vi "VisualizeWfrm.vi"() -> ()   [LabVIEW 2014, in "Visualization.lvlib" / "VisualizeWfrm.lvclass"]
uses:
  VisualizeWfrm.lvclass
  VisualizeBase/VisualizeBase_class/Requests/clUserEventType.ctl
  <vilib>/event_ctls.llb/usereventprio.ctl
  <vilib>/Utility/error.llb/Error Cluster From Error Code.vi
  <vilib>/ErrorRing/Error Ring.xnode
  VisualizeBase/VisualizeBase_class/VisualizeBase.lvclass
  <userlib>/NIST/NISTErrorLib/NISTErrorLib.lvlib
  WfrmGenerator/WfrmModule/WfrmModule.lvlib
panel:
  out "Currents":dbl[][](graph)
  out "Voltages":dbl[][](graph)
  in  "QueName":string="WfrmVisQue"
  out "ErrorArray":errorcluster[](array[cluster])
  in  "btnStop":bool
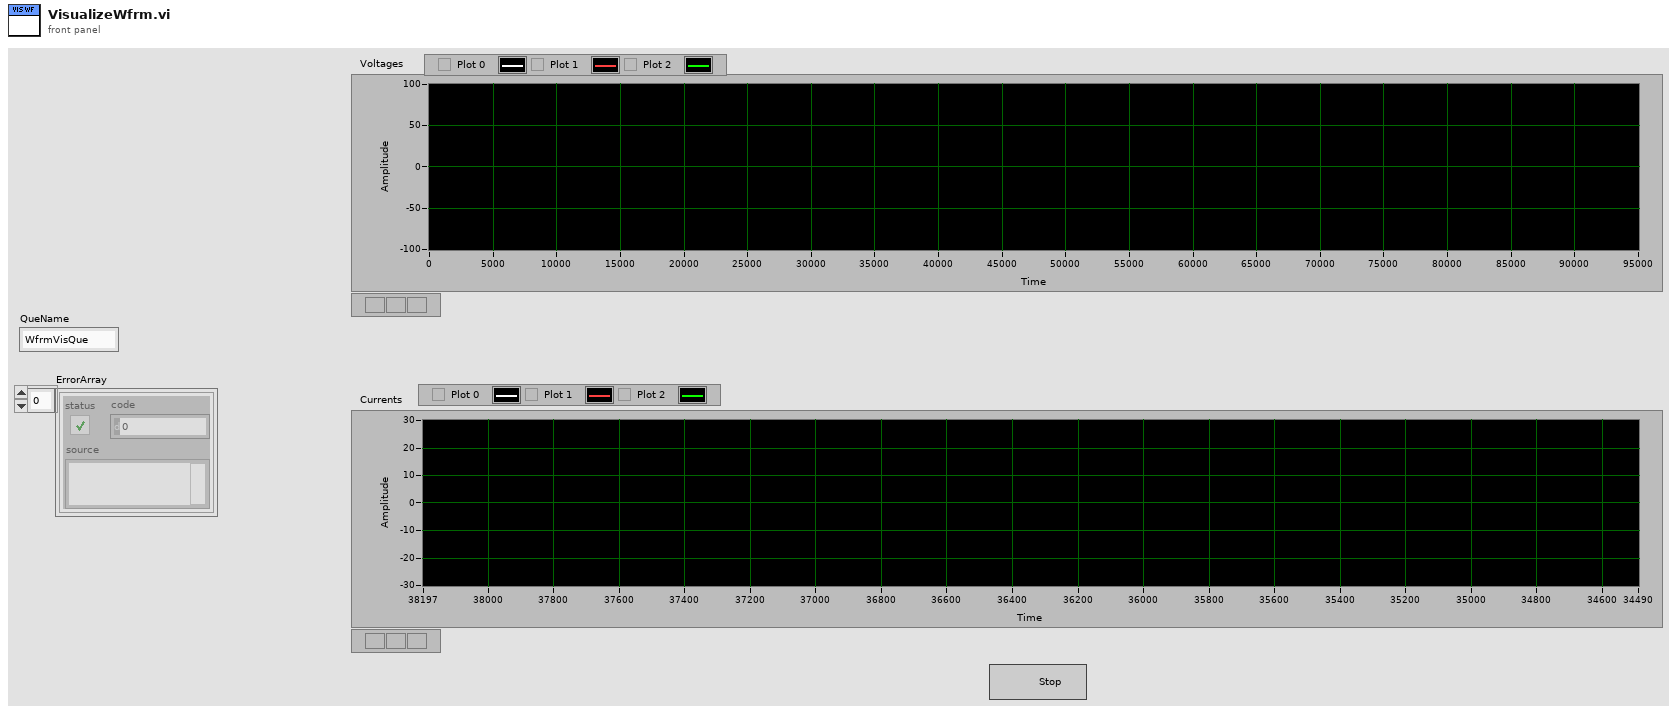
[diagram p1: front panel]
types:
  T1 = typedef "Visualization.lvlib/VisualizeBase.lvclass/clRequestEvents.ctl" = cluster{"StopRequest":refnum<user-event>}
  T2 = typedef "WfrmModule.lvlib/clBroadcastEvents.ctl" = cluster{"DidInit":refnum<user-event>, "StatusUpdate":refnum<user-event>, "ErrorReport":refnum<user-event>, "DidStop":refnum<user-event>, "ReadEvtConfig":refnum<user-event>, "ReadTimeArray":refnum<user-event>, "ReadEvtParams":refnum<user-event>, "GetEvtReportArray":refnum<user-event>, "ReadPathToPlugin":refnum<user-event>, "GetEvtSignal":refnum<user-event>, "SendArbWfrm":refnum<user-event>, "WfrmParams":refnum<user-event>}
  T3 = typedef "Visualization.lvlib/VisualizeBase.lvclass/clUserEventType.ctl" = cluster{"BusIndex":i8, "Data":variant}
  T4 = typedef "usereventprio.ctl" = enum32{"high priority", "normal priority"}
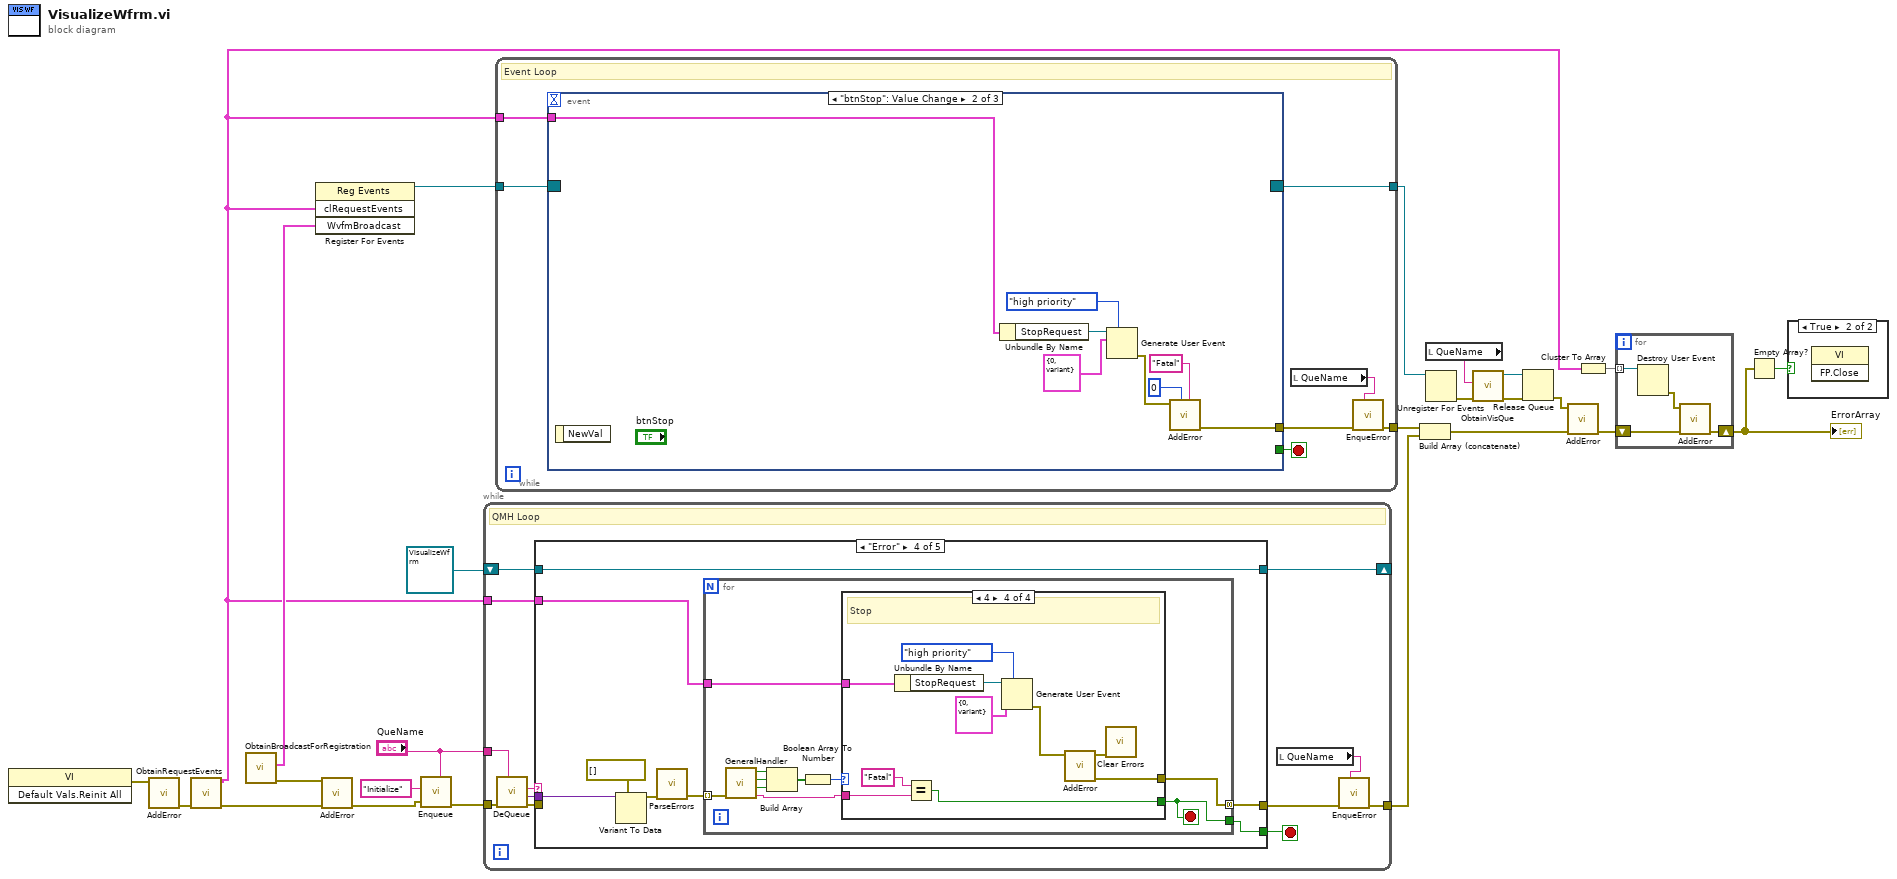
[diagram p0: block diagram]
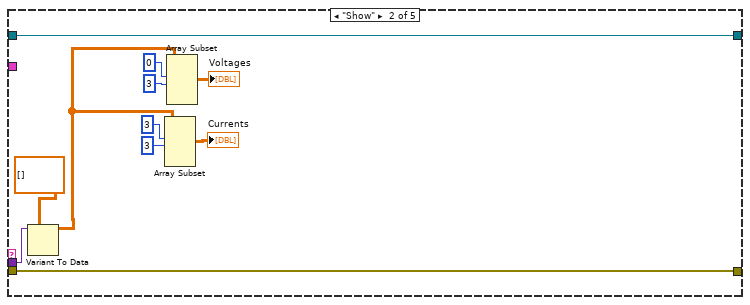
[diagram p4: hidden frame]
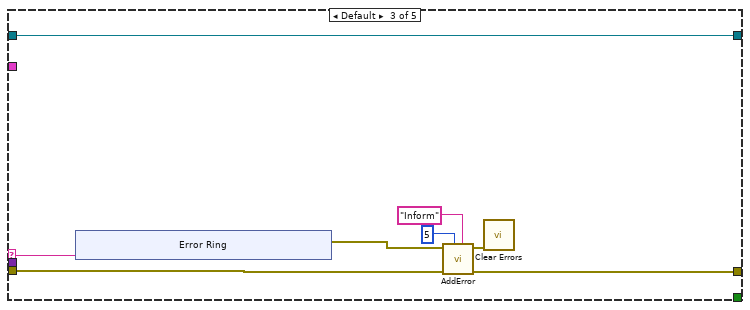
[diagram p5: hidden frame]
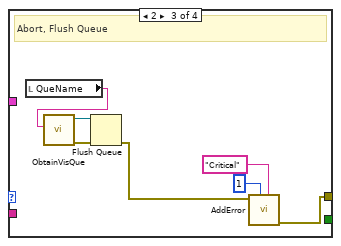
[diagram p8: hidden frame]
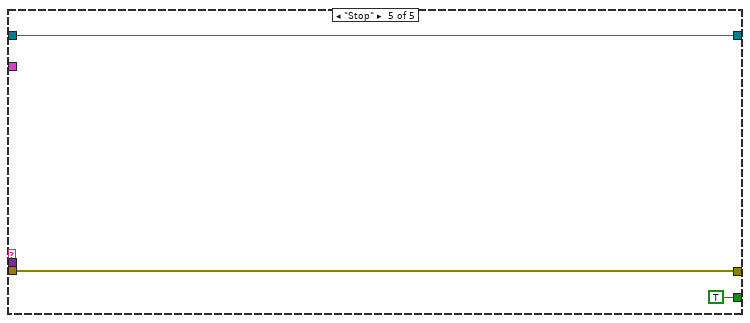
[diagram p9: hidden frame]
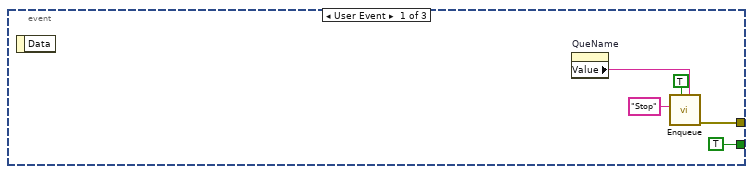
[diagram p10: hidden frame]
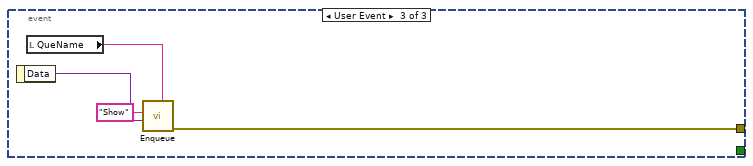
[diagram p11: hidden frame]
diagram:
  n1 = invoke class="VI" method="Default Vals.Reinit All"() -> (error out=w20:errorcluster)  [unwired: 3 in, 2 out]
  n2 = call <userlib>:"AddError.vi"("error in (no error)"=w20) -> ("ErrorArray"=w19:errorcluster[])  [unwired: 9 in, 1 out]
  n3 = call "ObtainRequestEvents.vi"("Error"=w19) -> ("Error"=w16:errorcluster[], "clRequestEvents"=w1:T1)  [unwired: 9 in]
  n4 = call "ObtainBroadcastForRegistration.vi"() -> ("error out"=w14:errorcluster, "WvfmBroadcast"=w17:T2)  [unwired: 10 in]
  n5 = register-events(w1, w17) -> (reference out=w23:refnum<event-registration>)  [unwired: 2 in, 1 out]
  n6 = call <userlib>:"AddError.vi"("ErrorArray"=w16, "error in (no error)"=w14) -> ("ErrorArray"=w15:errorcluster[])  [unwired: 8 in, 1 out]
  n7 = call "Enqueue.vi"("QueName"="QueName", "Error"=w15, "Message"="Initialize") -> ("Error"=w24:errorcluster[])  [unwired: 8 in]
  n8 = while {
    tunnel: w24 -> [w37]
    tunnel: [w31] -> w22
    tunnel: "QueName" -> [w29]
    shift-right: [w28] -> _
    shift-left: refnum<class "VisualizeWfrm.lvclass"> refnum ("VisualizeBase_class.lvclass") -> [w27]
    tunnel: w1 -> [w26]
    stop <- w32 stop-if-true
    # "QMH Loop"
    n9 = call "DeQueue.vi"("QueName"=w29, "Error"=w37) -> ("Error"=w34:errorcluster[], "Data"=w35:variant, "Message"=w36:string)  [unwired: 7 in]
    n10 = case shown="\"Error\"" w36 {
      selector: w36 -> [_ _ w58 _ _]
      tunnel: w35 -> [_ w48 _ w73 _]
      tunnel: w34 -> [w39 w50 w56 _ w102]
      tunnel: [w39 w50 w55 w69 w102] -> w33
      tunnel: [_ _ _ w68 TRUE] -> w32
      tunnel: w27 -> [w38 w49 w51 w67 w101]
      tunnel: [w38 w49 w51 w67 w101] -> w28
      tunnel: w26 -> [_ _ _ w66 _]
      frame "Initialize" {
      }
      frame "Show" {
        n11 = Variant To Data(type=dbl[][] [], Variant=w48) -> (data=w41:dbl[][])  [unwired: 1 in, 1 out]
        n12 = Array Subset(array=w41, index (row)=3 ("index"), length (row)=3 ("length")) -> (→"Currents":dbl[][])  [unwired: 2 in]
        n13 = Array Subset(array=w41, index (row)=0 ("index"), length (row)=3 ("length")) -> (→"Voltages":dbl[][])  [unwired: 2 in]
      }
      frame Default {
        n14 = xnode "Error Ring"("parameter 0"=w58) -> ("error out"=w57:errorcluster)
        n15 = call <userlib>:"AddError.vi"("Severity"="Inform" ("String"), "Priority"=u8 5, "ErrorArray"=w56, "error in (no error)"=w57) -> ("ErrorArray"=w55:errorcluster[], "error out"=w54:errorcluster)  [unwired: 6 in]
        n16 = call <vilib>:"Clear Errors.vi"("error in (no error)"=w54) -> ()  [unwired: 5 in, 2 out]
      }
      frame "Error" {
        n17 = Variant To Data(type=errorcluster[] [], Variant=w73) -> (data=w71:errorcluster[])  [unwired: 1 in, 1 out]
        n18 = call <userlib>:"ParseErrors.vi"("ErrorArray"=w71) -> ("ErrorArray"=w70:errorcluster[])  [unwired: 8 in, 2 out]
        n19 = for {
          tunnel: w70 -> [w83] mode=indexing
          tunnel: [w77] -> w69 mode=concatenating
          tunnel: [w75] -> w68
          tunnel: w66 -> [w74]
          stop <- w75 stop-if-true
          n20 = call <userlib>:"GeneralHandler.vi"("error in (no error)"=w83) -> ("Severity"=w76:string, "Stop"=w80:bool, "Abort"=w81:bool, "Continue"=w82:bool)  [unwired: 7 in]
          n21 = Build Array(w82, w81, w80) -> (w79:bool[])
          n22 = Boolean Array To Number(Boolean array=w79) -> (number=w78:u32)
          n23 = case shown="4" w78 {
            tunnel: [_ _ w88 w99] -> w77
            tunnel: w76 -> [_ _ _ w94]
            tunnel: [_ _ _ w92] -> w75
            tunnel: w74 -> [_ _ _ w91]
            frame 0, Default {
              # "No Dialog"
            }
            frame 1 {
              # "Continue"
            }
            frame 2 {
              # "Abort, Flush Queue"
              n24 = local read "QueName"() -> (w84:string)
              n25 = call "ObtainVisQue.vi"("QueName"=w84) -> ("error out"=w90:errorcluster, "queue out"=w89:refnum<queue>)  [unwired: 9 in]
              n26 = Flush Queue(queue=w89, error in (no error)=w90) -> (error out=w87:errorcluster)  [unwired: 2 out]
              n27 = call <userlib>:"AddError.vi"("Severity"="Critical" ("String"), "Priority"=u8 1, "error in (no error)"=w87) -> ("ErrorArray"=w88:errorcluster[])  [unwired: 7 in, 1 out]
            }
            frame 4 {
              # "Stop"
              n28 = Unbundle By Name(w91) -> ("StopRequest"=w100:refnum<user-event>)
              n29 = Equal?(x="Fatal", y=w94) -> (x = y?=w92:bool)
              n30 = Generate User Event(priority (normal)=usereventprio."high priority", user event=w100, event data cluster=T3 {"BusIndex"=0, "Data"=variant} ("event data")) -> (error out=w98:errorcluster)  [unwired: 1 in, 1 out]
              n31 = call <userlib>:"AddError.vi"("error in (no error)"=w98) -> ("ErrorArray"=w99:errorcluster[], "error out"=w95:errorcluster)  [unwired: 9 in]
              n32 = call <vilib>:"Clear Errors.vi"("error in (no error)"=w95) -> ()  [unwired: 5 in, 2 out]
            }
          }
        }
      }
      frame "Stop" {
      }
    }
    n33 = local read "QueName"() -> (w30:string)
    n34 = call "EnqueError.vi"("QueName"=w30, "Error"=w33) -> ("Error"=w31:errorcluster[])  [unwired: 9 in]
  }
  n35 = while {
    tunnel: w23 -> [w110]
    tunnel: [w107] -> w21
    tunnel: w1 -> [w105]
    tunnel: [w104] -> w9
    stop <- w109 stop-if-true
    # "Event Loop"
    n36 = event shown="[1] \"btnStop\": Value Change" {
      selector: w110 -> [_ _ _]
      dyn-events: [_ _ _] -> w104
      timeout: _ -> [_ _ _]
      tunnel: [TRUE _ _] -> w109
      tunnel: [w114 w121 w125] -> w108
      tunnel: w105 -> [_ w116 _]
      event User Event {
        n37 = event-data() -> ()  [unwired: 1 in, 1 out]
        n38 = property on="QueName" class="Str"() -> ("Value"=w111:string)  [unwired: 2 in, 2 out]
        n39 = call "Enqueue.vi"("QueName"=w111, "Priority? (F)"=TRUE, "Message"="Stop") -> ("Error"=w114:errorcluster[])  [unwired: 8 in]
      }
      event "btnStop": Value Change {
        n40 = event-data() -> ()  [unwired: 1 in, 1 out]
        n41 = Unbundle By Name(w116) -> ("StopRequest"=w122:refnum<user-event>)
        n42 = Generate User Event(priority (normal)=usereventprio."high priority", user event=w122, event data cluster=T3 {"BusIndex"=0, "Data"=variant} ("event data")) -> (error out=w123:errorcluster)  [unwired: 1 in, 1 out]
        n43 = call <userlib>:"AddError.vi"("Severity"="Fatal" ("String"), "Priority"=u8 0, "error in (no error)"=w123) -> ("ErrorArray"=w121:errorcluster[])  [unwired: 7 in, 1 out]
      }
      event User Event {
        n44 = event-data() -> ("Data"=w126:variant)  [unwired: 1 in]
        n45 = local read "QueName"() -> (w127:string)
        n46 = call "Enqueue.vi"("QueName"=w127, "Data"=w126, "Message"="Show") -> ("Error"=w125:errorcluster[])  [unwired: 8 in]
      }
    }
    n47 = local read "QueName"() -> (w106:string)
    n48 = call "EnqueError.vi"("QueName"=w106, "Error"=w108) -> ("Error"=w107:errorcluster[])  [unwired: 9 in]
  }
  n49 = Build Array (concatenate)(w21, w22) -> (w8:errorcluster[])
  n50 = local read "QueName"() -> (w10:string)
  n51 = Unregister For Events(event registration refnum=w9) -> (error out=w11:errorcluster)  [unwired: 1 in]
  n52 = call "ObtainVisQue.vi"("error in (no error)"=w11, "QueName"=w10) -> ("error out"=w12:errorcluster, "queue out"=w2:refnum<queue>)  [unwired: 8 in]
  n53 = Release Queue(queue=w2, error in (no error)=w12) -> (error out=w7:errorcluster)  [unwired: 1 in, 2 out]
  n54 = call <userlib>:"AddError.vi"("ErrorArray"=w8, "error in (no error)"=w7) -> ("ErrorArray"=w5:errorcluster[])  [unwired: 8 in, 1 out]
  n55 = Cluster To Array(cluster=w1) -> (array=w6:refnum<user-event>[])
  n56 = for {
    tunnel: w6 -> [w131] mode=indexing
    shift-right: [w130] -> w3
    shift-left: w5 -> [w129]
    n57 = Destroy User Event(user event=w131) -> (error out=w128:errorcluster)  [unwired: 1 in]
    n58 = call <userlib>:"AddError.vi"("ErrorArray"=w129, "error in (no error)"=w128) -> ("ErrorArray"=w130:errorcluster[])  [unwired: 8 in, 1 out]
  }
  "ErrorArray" <- w3
  n59 = Empty Array?(array=w3) -> (empty?=w4:bool)
  n60 = case shown="True" w4 {
    frame False {
    }
    frame True {
      n61 = invoke class="VI" method="FP.Close"() -> ()  [unwired: 3 in, 3 out]
    }
  }
